vi "Format 2D Array for Save.vi"(8 "error in (no error)":errorcluster, 11 "Signals":string[][](array[string])) -> (0 "error out":errorcluster, 3 "Formated Table":string[][](array[string]))   [LabVIEW 2025, in "Project.lvclass"]
uses:
  Project.lvclass
panel:
  out "element":i32
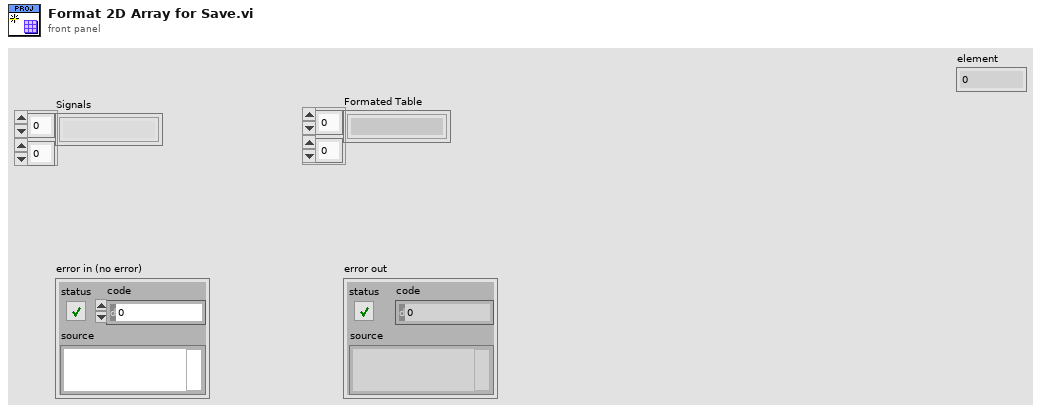
[diagram p1: front panel]
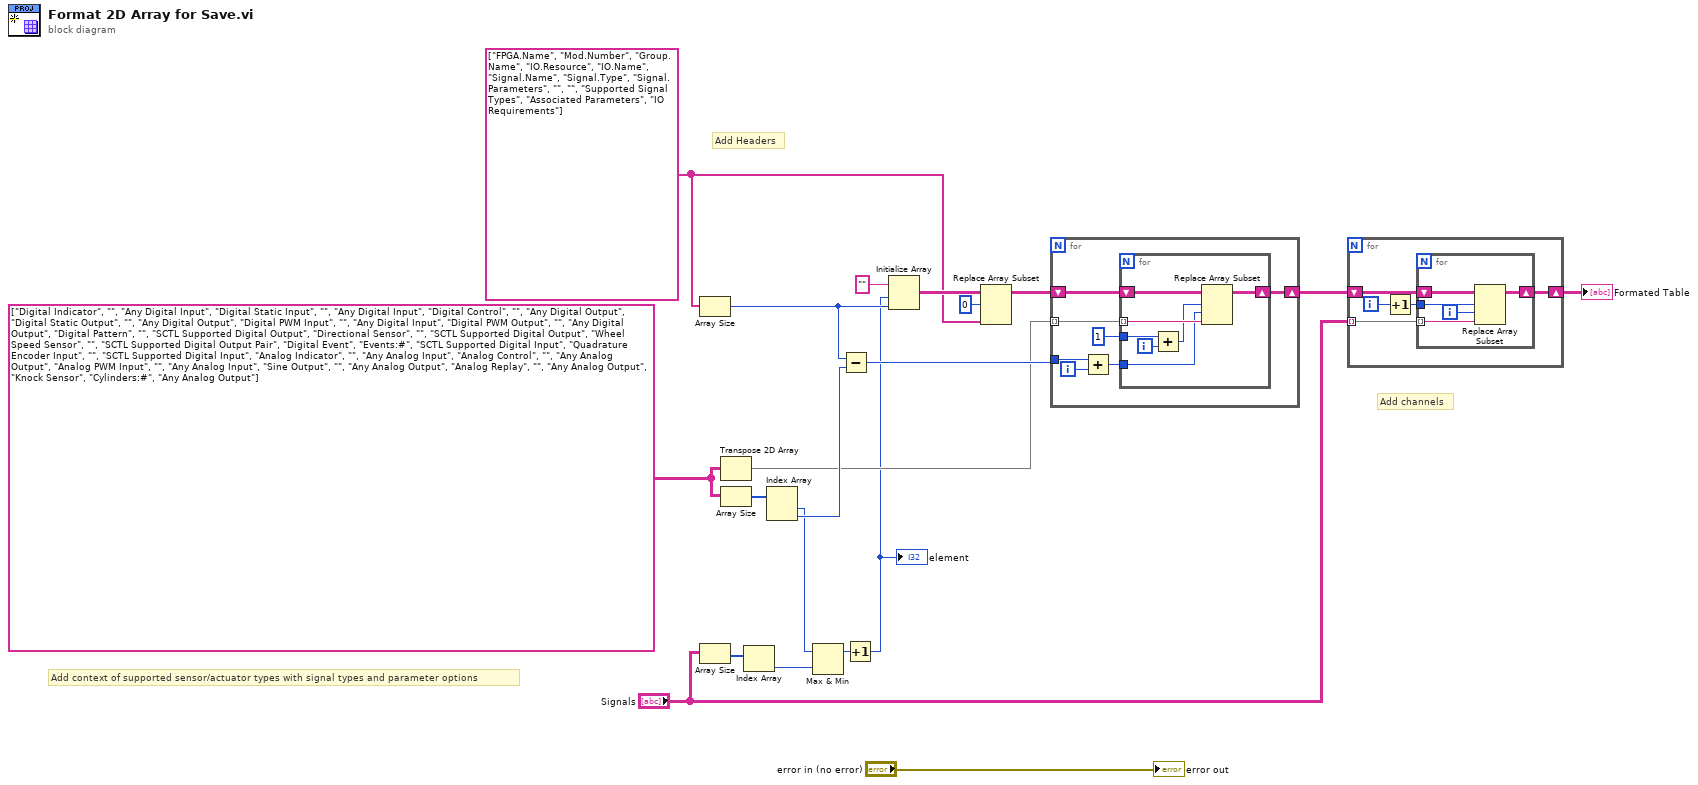
[diagram p0: block diagram]
diagram:
  w5 = string[] ["FPGA.Name", "Mod.Number", "Group.Name", "IO.Resource", "IO.Name", "Signal.Name", "Signal.Type", "Signal.Parameters", "", "", "Supported Signal Types", "Associated Parameters", "IO Requirements"] ("names")
  w11 = string[][] [["Digital Indicator", "", "Any Digital Input"], ["Digital Static Input", "", "Any Digital Input"], ["Digital Control", "", "Any Digital Output"], ["Digital Static Output", "", "Any Digital Output"], ["Digital PWM Input", "", "Any Digital Input"], ["Digital PWM Output", "", "Any Digital Output"], ["Digital Pattern", "", "SCTL Supported Digital Output"], ["Directional Sensor", "", "SCTL Supported Digital Output"], ["Wheel Speed Sensor", "", "SCTL Supported Digital Output Pair"], ["Digital Event", "Events:#", "SCTL Supported Digital Input"], ["Quadrature Encoder Input", "", "SCTL Supported Digital Input"], ["Analog Indicator", "", "Any Analog Input"], ["Analog Control", "", "Any Analog Output"], ["Analog PWM Input", "", "Any Analog Input"], ["Sine Output", "", "Any Analog Output"], ["Analog Replay", "", "Any Analog Output"], ["Knock Sensor", "Cylinders:#", "Any Analog Output"]] ("Array")
  # "Add channels"
  # "Add context of supported sensor/actuator types with signal types and parameter options"
  # "Add Headers"
  n1 = Array Size(array=w5) -> (size(s)=w9:i32)
  n2 = Array Size(array="Signals") -> (size(s)=w18:i32[])
  n3 = Transpose 2D Array(2D array=w11) -> (transposed array=w10:string[][])
  n4 = Array Size(array=w11) -> (size(s)=w20:i32[])
  n5 = Index Array(array=w18) -> (element=w3:i32)  [unwired: 1 in]
  n6 = Index Array(array=w20) -> (element #1=w2:i32, element #2=w13:i32)  [unwired: 2 in]
  n7 = Max & Min(x=w2, y=w3) -> (max(x,y)=w17:i32)  [unwired: 1 out]
  n8 = Subtract(x=w9, y=w13) -> (x-y=w12:i32)
  n9 = Increment(x=w17) -> (x+1=w1:i32)
  "element" <- w1
  n10 = Initialize Array("", w1, w9) -> (w16:string[][])
  n11 = Replace Array Subset(array=w16, new element=w5, index (row)=0) -> (w14:string[][])  [unwired: 1 in]
  n12 = for {
    tunnel: w12 -> [w26]
    tunnel: w10 -> [w25] mode=indexing
    shift-right: [w22] -> w8
    shift-left: w14 -> [w27]
    i -> [w23]
    n13 = Add(x=w26, y=w23) -> (x+y=w24:i32)
    n14 = for {
      tunnel: w25 -> [w33] mode=indexing
      tunnel: w24 -> [w32]
      tunnel: 1 ("disabled index (row)") -> [w30]
      shift-right: [w31] -> w22
      shift-left: w27 -> [w34]
      i -> [w28]
      n15 = Add(x=w30, y=w28) -> (x+y=w29:i32)
      n16 = Replace Array Subset(array=w34, new element=w33, index (row)=w29, index (col)=w32) -> (w31:string[][])
    }
  }
  n17 = for {
    tunnel: "Signals" -> [w38] mode=indexing
    shift-right: [w37] -> w7
    shift-left: w8 -> [w39]
    i -> [w36]
    n18 = Increment(x=w36) -> (x+1=w35:i32)
    n19 = for {
      tunnel: w38 -> [w43] mode=indexing
      shift-right: [w42] -> w37
      shift-left: w39 -> [w44]
      tunnel: w35 -> [w40]
      i -> [w41]
      n20 = Replace Array Subset(array=w44, new element=w43, index (row)=w40, index (col)=w41) -> (w42:string[][])
    }
  }
  "Formated Table" <- w7
  "error out" <- "error in (no error)"
